vi "ManageDAQ.vi"(8 "error in":errorcluster, 9 "StreamTypeDef":T1, 10 "data type":variant, 11 "index":i32) -> (0 "error out":errorcluster, 1 "StreamTypeDef":T1, 3 "Index+1":i32)   [LabVIEW 2024]
uses:
  Control/StreamTypeDef.ctl
  Control/streamIO_states.ctl
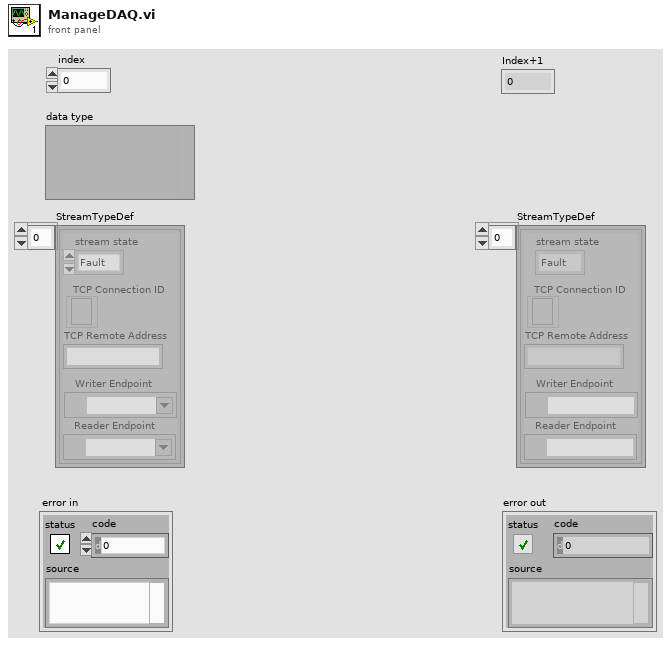
[diagram p1: front panel]
types:
  T1 = typedef "StreamTypeDef.ctl" = cluster{"stream state":T2, "TCP Remote Address":string, "TCP Connection ID":refnum<k5>, "Reader Endpoint":refnum<k21>, "Writer Endpoint":refnum<k21>}[]
  T2 = typedef "streamIO_states.ctl" = enum16{"Fault", "Initilize", "Stream", "Close"}
  T3 = cluster{"stream state":T2, "TCP Remote Address":string, "TCP Connection ID":refnum<k5>, "Reader Endpoint":refnum<k21>, "Writer Endpoint":refnum<k21>}
  T4 = enum16{"Standard", "Buffered", "CRLF", "Immediate"}
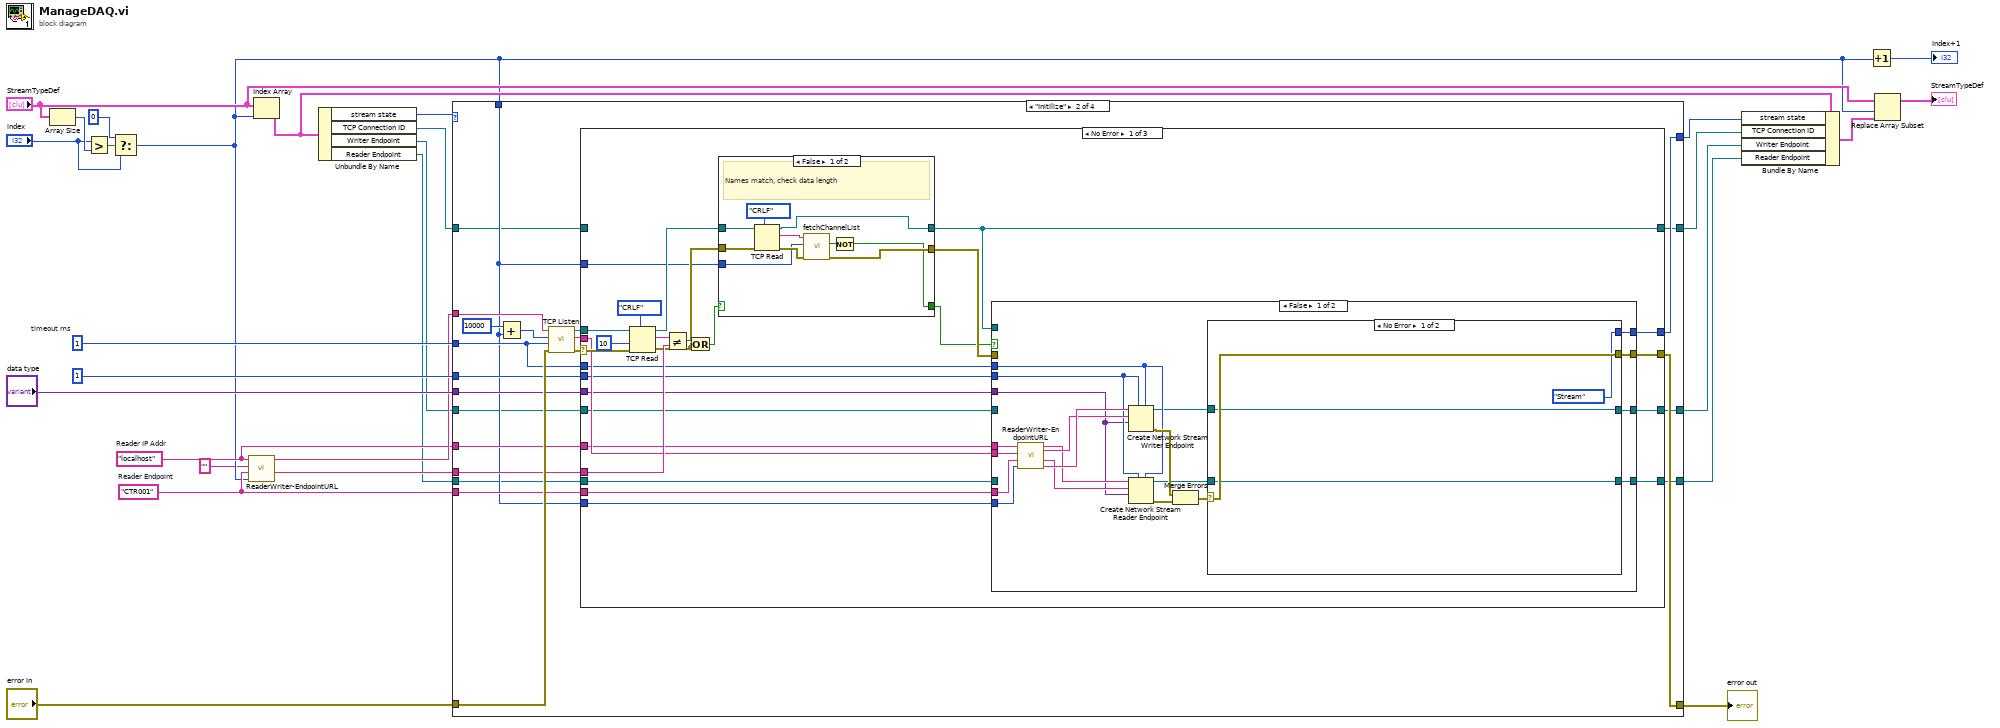
[diagram p0: block diagram]
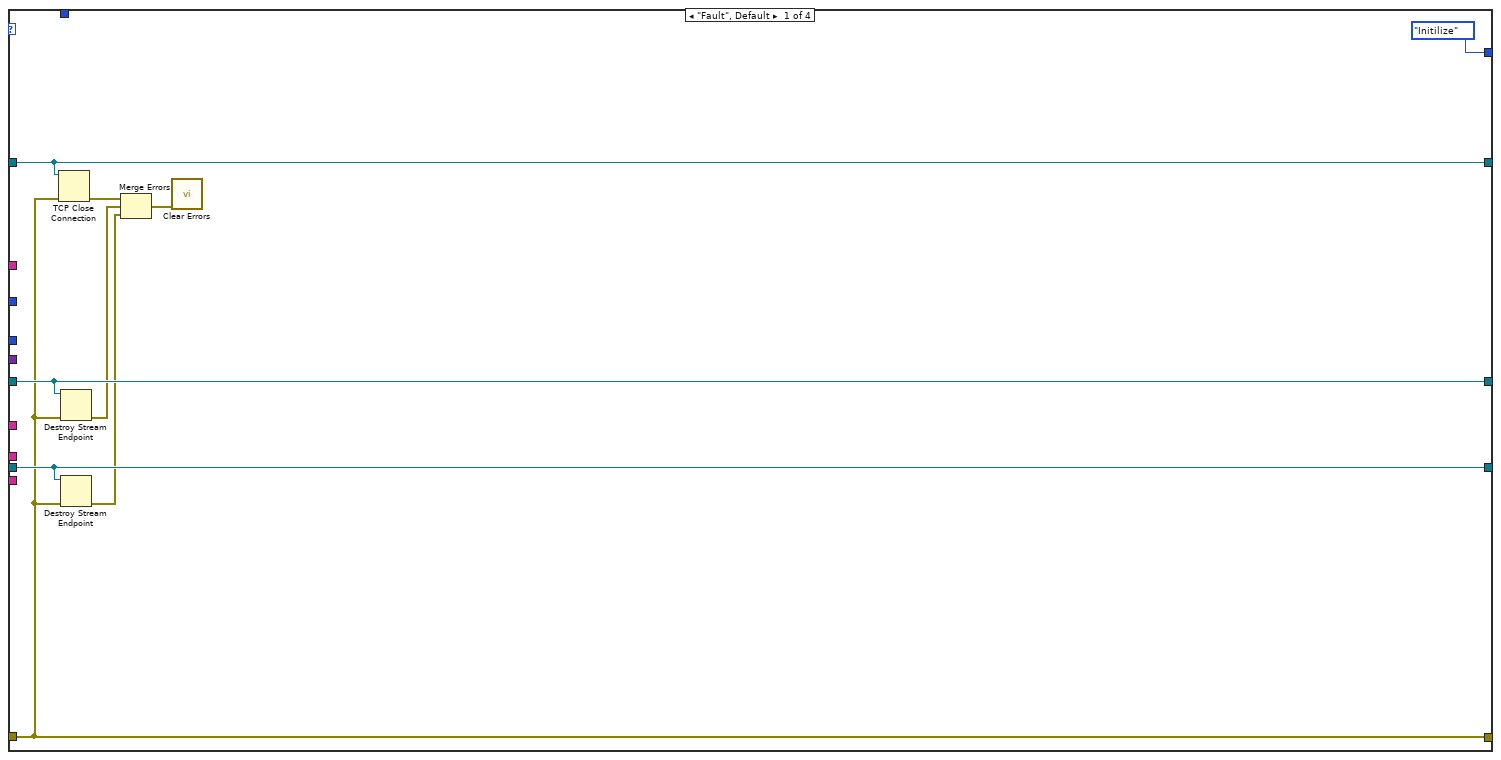
[diagram p2: hidden frame]
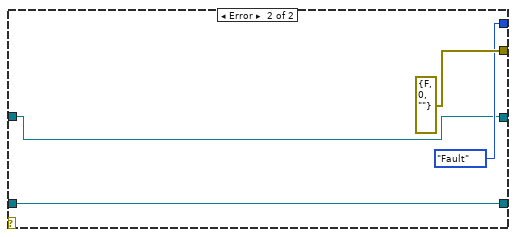
[diagram p4: hidden frame]
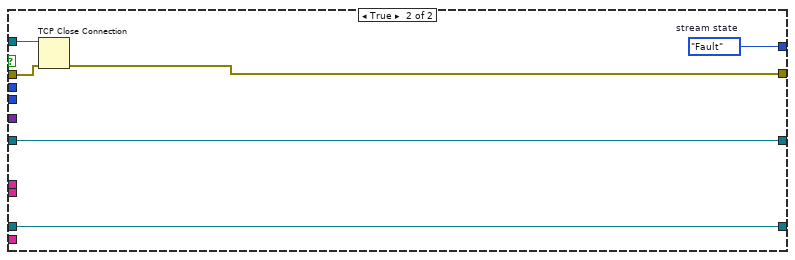
[diagram p5: hidden frame]
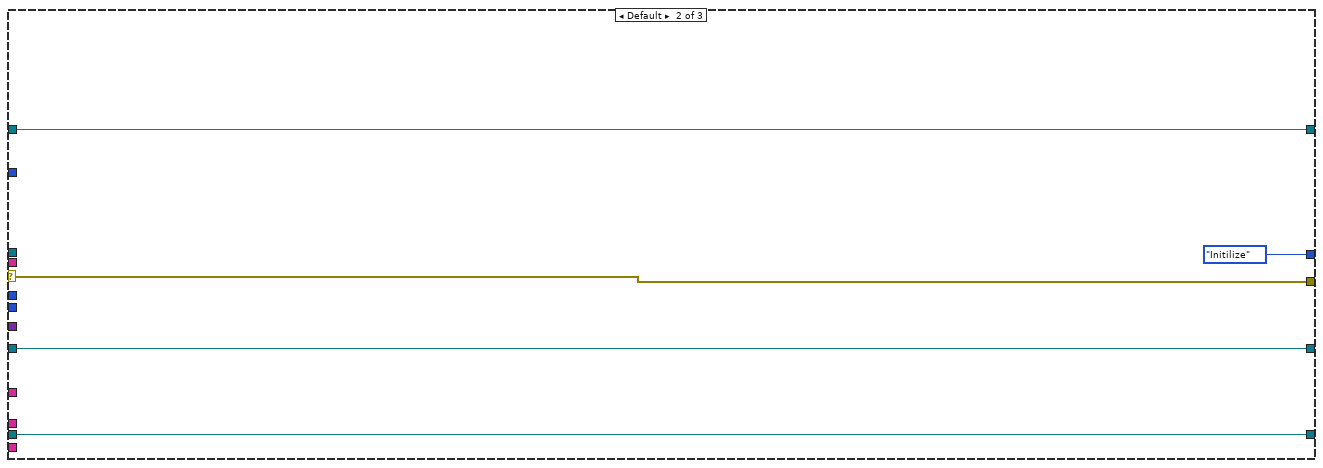
[diagram p6: hidden frame]
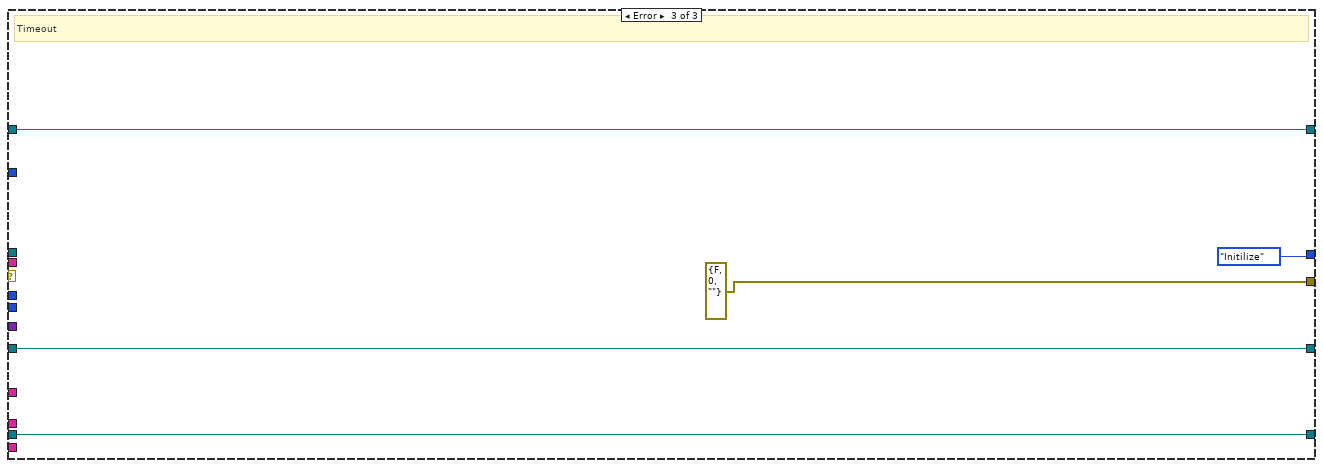
[diagram p7: hidden frame]
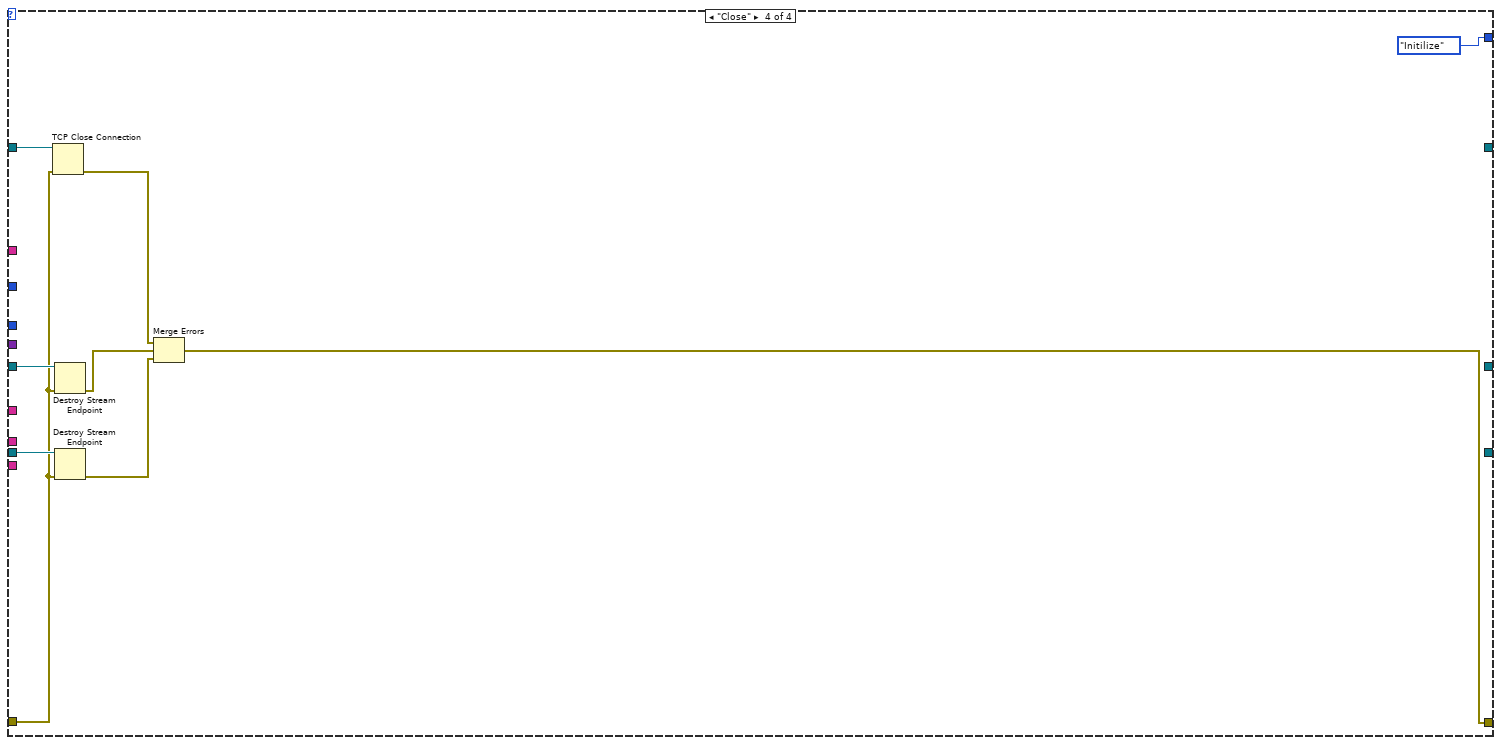
[diagram p9: hidden frame]
diagram:
  w22 = "localhost"  # Reader IP Addr
  w21 = "CTR001"  # Reader Endpoint
  w27 = 1  # timeout ms
  n1 = Array Size(array="StreamTypeDef") -> (size(s)=w20:i32)
  n2 = Greater?(x="index", y=w20) -> (0:w19:bool)
  n3 = Select(t=0, s=w19, f="index") -> (s? t:f=w10:i32)
  n4 = call "ReaderWriter-EndpointURL.vi"("DAQ ID #"=w10, "CTR Endpoint"=w21, "DAQ IR Addr"="", "CTR IP Addr"=w22) -> ("DAQ Endpoint"=w23:string, "CTR URL"=w24:string)  [unwired: 4 in, 2 out]
  n5 = Index Array(array="StreamTypeDef", index=w10) -> (element=w14:T3)
  n6 = Unbundle By Name(w14) -> ("stream state"=w15:T2, "TCP Connection ID"=w5:refnum<k5>, "Writer Endpoint"=w2:refnum<k21>, "Reader Endpoint"=w1:refnum<k21>)
  n7 = case shown="\"Initilize\"" w15 {
    selector: w15 -> [_ _ w144 _]
    tunnel: [streamIO_states."Initilize" ("Enum") w51 w144 streamIO_states."Initilize" ("Enum")] -> w13
    tunnel: "error in" -> [w34 w59 w145 w150]
    tunnel: w27 -> [_ w46 _ _]
    tunnel: [w34 w57 w145 w146] -> w7
    tunnel: w24 -> [_ w56 _ _]
    tunnel: w23 -> [_ w52 _ _]
    tunnel: w22 -> [_ w49 _ _]
    tunnel: w21 -> [_ w48 _ _]
    tunnel: 1 -> [_ w47 _ _]
    tunnel: "data type" -> [_ w45 _ _]
    tunnel: w10 -> [_ w44 _ _]
    tunnel: [w33 w43 _ _] -> w6
    tunnel: w5 -> [w33 w42 _ w151]
    tunnel: [w35 w41 _ _] -> w3
    tunnel: [w36 w40 _ _] -> w4
    tunnel: w2 -> [w35 w39 _ w152]
    tunnel: w1 -> [w36 w38 _ w153]
    frame "Fault", Default {
      n8 = TCP Close Connection(connection ID=w33, error in (no error)=w34) -> (error out=w32:errorcluster)  [unwired: 1 in, 1 out]
      n9 = Destroy Stream Endpoint(8:w34, 11:w35) -> (0:w31:errorcluster)
      n10 = Destroy Stream Endpoint(8:w34, 11:w36) -> (0:w30:errorcluster)
      n11 = Merge Errors(w32, w31, w30) -> (w29:errorcluster)
      n12 = call <vilib>:"Clear Errors.vi"("error in (no error)"=w29) -> ()  [unwired: 5 in, 2 out]
    }
    frame "Initilize" {
      n13 = Add(x=u16 10000 ("port"), y=w44) -> (x+y=w54:i32)
      n14 = call <vilib>:"TCP Listen.vi"("error in (no error)"=w59, "timeout ms (wait forever: -1)"=w46, "port"=w54, "service name"=w56) -> ("error out"=w58:errorcluster, "remote address"=w50:string, "connection ID"=w53:refnum<k5>)  [unwired: 3 in, 2 out]
      n15 = case shown="No Error" w58 {
        selector: w58 -> [w85 w138 _]
        tunnel: [w79 w138 errorcluster {"status"=FALSE, "code"=0, "source"=""} ("error IO")] -> w57
        tunnel: w53 -> [w84 _ _]
        tunnel: w52 -> [w82 _ _]
        tunnel: [w78 streamIO_states."Initilize" ("stream state") streamIO_states."Initilize" ("stream state")] -> w51
        tunnel: w50 -> [w77 _ _]
        tunnel: w49 -> [w76 _ _]
        tunnel: w48 -> [w75 _ _]
        tunnel: w44 -> [w74 _ _]
        tunnel: w47 -> [w73 _ _]
        tunnel: w46 -> [w72 _ _]
        tunnel: w45 -> [w71 _ _]
        tunnel: w44 -> [w65 _ _]
        tunnel: [w64 w136 w141] -> w43
        tunnel: w42 -> [_ w136 w141]
        tunnel: [w63 w135 w140] -> w41
        tunnel: [w62 w134 w139] -> w40
        tunnel: w39 -> [w61 w135 w140]
        tunnel: w38 -> [w60 w134 w139]
        frame No Error {
          n16 = TCP Read(connection ID=w84, error in (no error)=w85, 7:T4."CRLF" ("mode (standard)"), 9:10 ("timeout ms (25000)")) -> (connection ID out=w69:refnum<k5>, data out=w81:string, error out=w68:errorcluster)  [unwired: 1 in]
          n17 = Not Equal?(x=w81, y=w82) -> (x != y?=w80:bool)
          n18 = Or(x=w80, y=w68) -> (x .or. y?=w70:bool)
          n19 = case shown="False" w70 {
            selector: w70 -> [_ w99]
            tunnel: [w88 w99] -> w66
            tunnel: w69 -> [w96 w98]
            tunnel: [w87 w98] -> w64
            tunnel: w68 -> [w95 w97]
            tunnel: [w92 w97] -> w67
            tunnel: w65 -> [w90 _]
            frame False {
              # "Names match, check data length"
              n20 = TCP Read(connection ID=w96, error in (no error)=w95, 7:T4."CRLF" ("mode (standard)")) -> (connection ID out=w87:refnum<k5>, data out=w91:string, error out=w93:errorcluster)  [unwired: 2 in]
              n21 = call "fetchChannelList.vi"("error in"=w93, "DAQ ID #"=w90, "Channels"=w91) -> ("error out"=w92:errorcluster, "Channel Match?"=w89:bool)  [unwired: 6 in, 1 out]
              n22 = Not(x=w89) -> (.not. x?=w88:bool)
            }
            frame True {
              # "names not equal, abort"
            }
          }
          n23 = case shown="False" w66 {
            tunnel: w64 -> [_ w133]
            tunnel: w67 -> [_ w132]
            tunnel: [w116 w131] -> w79
            tunnel: [w115 w130] -> w78
            tunnel: w77 -> [w114 _]
            tunnel: w76 -> [w113 _]
            tunnel: w75 -> [w112 _]
            tunnel: w74 -> [w111 _]
            tunnel: w73 -> [w106 _]
            tunnel: w72 -> [w105 _]
            tunnel: w71 -> [w104 _]
            tunnel: [w102 w129] -> w63
            tunnel: [w101 w128] -> w62
            tunnel: w61 -> [_ w129]
            tunnel: w60 -> [_ w128]
            frame False {
              n24 = call "ReaderWriter-EndpointURL.vi"("DAQ ID #"=w111, "CTR Endpoint"=w112, "DAQ IR Addr"=w114, "CTR IP Addr"=w113) -> ("CTR Endpoint"=w110:string, "DAQ Endpoint"=w107:string, "DAQ URL"=w109:string, "CTR URL"=w108:string)  [unwired: 4 in]
              n25 = Create Network Stream Writer Endpoint(5:w105, 7:w106, 9:w104, 10:w109, 11:w110) -> (0:w117:errorcluster, 3:w103:refnum<k21>)  [unwired: 2 in]
              n26 = Create Network Stream Reader Endpoint(5:w105, 7:w106, 9:w104, 10:w107, 11:w108) -> (0:w118:errorcluster, 3:w100:refnum<k21>)  [unwired: 2 in]
              n27 = Merge Errors(w117, w118) -> (w119:errorcluster)
              n28 = case shown="No Error" w119 {
                selector: w119 -> [w123 _]
                tunnel: [w123 errorcluster {"status"=FALSE, "code"=0, "source"=""} ("error IO")] -> w116
                tunnel: [streamIO_states."Stream" ("stream state") streamIO_states."Fault" ("stream state")] -> w115
                tunnel: [w121 w125] -> w102
                tunnel: w103 -> [w121 w125]
                tunnel: [w120 w124] -> w101
                tunnel: w100 -> [w120 w124]
                frame No Error {
                }
                frame Error {
                }
              }
            }
            frame True {
              w130 = streamIO_states."Fault"  # stream state
              n29 = TCP Close Connection(connection ID=w133, error in (no error)=w132) -> (error out=w131:errorcluster)  [unwired: 1 in, 1 out]
            }
          }
        }
        frame Default {
        }
        frame Error {
          # "Timeout"
        }
      }
    }
    frame "Stream" {
    }
    frame "Close" {
      n30 = TCP Close Connection(connection ID=w151, error in (no error)=w150) -> (error out=w147:errorcluster)  [unwired: 1 in, 1 out]
      n31 = Destroy Stream Endpoint(8:w150, 11:w152) -> (0:w148:errorcluster)
      n32 = Destroy Stream Endpoint(8:w150, 11:w153) -> (0:w149:errorcluster)
      n33 = Merge Errors(w147, w148, w149) -> (w146:errorcluster)
    }
  }
  "error out" <- w7
  n34 = Bundle By Name(cluster=w14, "stream state"=w13, "TCP Connection ID"=w6, "Writer Endpoint"=w3, "Reader Endpoint"=w4) -> (w12:T3)
  n35 = Increment(x=w10) -> (x+1=→"Index+1":i32)
  n36 = Replace Array Subset(array="StreamTypeDef", new element=w12, index=w10) -> (→"StreamTypeDef":T1)
